vi "Close in Callback Server.vi"() -> ()   [LabVIEW 2020, in "TCP Tests.lvlib"]
uses:
  TCP Tests.lvlib
  Stream-TCP/TCP Server/TCP Server.lvclass
  C:/Program Files (x86)/National Instruments/LabVIEW 2020/vi.lib/IlluminatedG/lv-stream/Endpoint/Endpoint.lvclass
  Close in Connection State Callback.vi
  <vilib>/IlluminatedG/lv-stream/Endpoint/Endpoint.lvclass
panel:
  in  "stop":bool
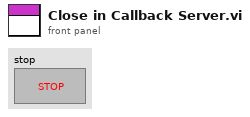
[diagram p1: front panel]
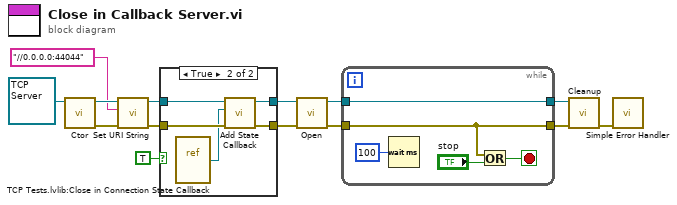
[diagram p0: block diagram]
diagram:
  n1 = call-dynamic "Ctor.vi"("TCP Server in"=refnum<class "TCP Server.lvclass"> refnum) -> ("error out"=w12:errorcluster, "TCP Server out"=w14:refnum<class "TCP Server.lvclass">)  [unwired: 9 in]
  n2 = call <vilib>:"Set URI String.vi"("error in (no error)"=w12, "URI String"="//0.0.0.0:44044", "Endpoint in"=w14) -> ("error out"=w5:errorcluster, "Endpoint out"=w4:refnum<class "TCP Server.lvclass">)  [unwired: 7 in]
  n3 = case shown="True" TRUE {
    tunnel: w5 -> [w15 w21]
    tunnel: w4 -> [w16 w20]
    tunnel: [w15 w19] -> w3
    tunnel: [w16 w18] -> w2
    frame False {
    }
    frame True {
      n4 = vi-ref "TCP Tests.lvlib:Close in Connection State Callback.vi"() -> (w17:refnum<vi>)
      n5 = call-dynamic "Add State Callback.vi"("error in (no error)"=w21, "Callback"=w17, "Endpoint in"=w20) -> ("error out"=w19:errorcluster, "Endpoint out"=w18:refnum<class "TCP Server.lvclass">)  [unwired: 7 in]
    }
  }
  n6 = call <vilib>:"Open.vi"("error in (no error)"=w3, "Endpoint in"=w2) -> ("error out"=w10:errorcluster, "Endpoint out"=w11:refnum<class "TCP Server.lvclass">)  [unwired: 8 in]
  n7 = while {
    tunnel: w11 -> [w22]
    tunnel: w10 -> [w23]
    tunnel: [w23] -> w8
    tunnel: [w22] -> w9
    stop <- w24 stop-if-true
    n8 = Wait (ms)(milliseconds to wait=u32 100) -> ()  [unwired: 1 out]
    n9 = Or(x=w23, y="stop") -> (x .or. y?=w24:bool)
  }
  n10 = call-dynamic "Cleanup.vi"("error in (no error)"=w8, "TCP Server in"=w9) -> ("error out"=w7:errorcluster)  [unwired: 9 in]
  n11 = call <vilib>:"Simple Error Handler.vi"("error in (no error)"=w7) -> ()  [unwired: 4 in, 5 out]
